vi "thrustAlloc.vi"(2 "tau":dbl[](array[numeric])) -> (5 "u_0":dbl, 6 "u_1":dbl, 7 "u_2":dbl)   [LabVIEW 2014]
uses:
  <vilib>/imath/engines/lvmath2/RunTimeEngine/Managers/WorkSpace/UID Generator.vi
  <vilib>/imath/engines/lvmath2/RunTimeEngine/ArithmeticOperatorToken/NIMS_ArithmeticOperator_multmx(M,CV).vi
  <instcachedir>/0/NIMS_ArithmeticOperator_multmx(M,CV)_787B4652E60B4C52835A7FB23671E425.lvgen/NIMS_ArithmeticOperator_multmx(M,CV)_787B4652E60B4C52835A7FB23671E425_000.vi
  <vilib>/imathl/engines/lvmath/Functions/Error Handling/Create Error.vi
  <vilib>/imath/engines/lvmath2/RunTimeEngine/IndexRead/NIMS M(S).vi
  <instcachedir>/0/NIMS M(S)_B826C018497E4940AE96BD27B540B6FB.lvgen/NIMS M(S)_B826C018497E4940AE96BD27B540B6FB_000.vi
  <vilib>/imath/engines/lvmath2/RunTimeEngine/BuiltInFunctions/diag/NIMS_diag.vi
  <instcachedir>/0/NIMS_diag_3C4F3DCE8A2D4541A558217542783B22.lvgen/NIMS_diag_3C4F3DCE8A2D4541A558217542783B22_003.vi
  <vilib>/imath/engines/lvmath2/RunTimeEngine/RunTimeType/NIMS_RunTimeType_From StrictType (excl LVString).vi
  <instcachedir>/0/NIMS_RunTimeType_From StrictType (excl LVString)_15A5391EEA9C4AACB9955AC755B83D29.lvgen/NIMS_RunTimeType_From StrictType (excl LVString)_15A5391EEA9C4AACB9955AC755B83D29_000.vi
  <vilib>/imath/engines/lvmath2/RunTimeEngine/LocalVariableDefStatement/MC_LocalVariableDefStatement_Display.vi
  <vilib>/imath/engines/lvmath2/RunTimeEngine/ArithmeticOperatorToken/NIMS_ArithmeticOperator_multmx.vi
  <instcachedir>/0/NIMS_ArithmeticOperator_multmx_CE3986B82B8C4E94A31593A7EF82383B.lvgen/NIMS_ArithmeticOperator_multmx_CE3986B82B8C4E94A31593A7EF82383B_004.vi
  <vilib>/imath/engines/lvmath2/RunTimeEngine/BuiltInFunctions/inv/NIMS_inv(GM).vi
  <instcachedir>/0/NIMS_inv(GM)_A6DF8FE880224208AACFE4CF9F659502.lvgen/NIMS_inv(GM)_A6DF8FE880224208AACFE4CF9F659502_000.vi
  <vilib>/imath/engines/lvmath2/RunTimeEngine/ErrorHandling/NIMS_Error From Error Code.vi
  <vilib>/imath/engines/lvmath2/RunTimeEngine/Managers/SymbolTable/Clear UID.vi
  <vilib>/imath/engines/lvmath2/RunTimeEngine/NodeEndStatement/NIMS_NodeEndStatement_Output.vi
  <instcachedir>/0/NIMS_NodeEndStatement_Output_53EC0D466D134D7ABD903AC30B43404B.lvgen/NIMS_NodeEndStatement_Output_53EC0D466D134D7ABD903AC30B43404B_002.vi
  <vilib>/imath/engines/lvmath2/RunTimeEngine/ErrorHandling/NIMS_Finalize Error.vi
  <vilib>/imath/engines/lvmath2/RunTimeEngine/ErrorHandling/NIMS_Create Error From Enums.vi
  <vilib>/imath/engines/lvmath2/RunTimeEngine/ArithmeticOperatorToken/NIMS_ArithmeticOperator_multmx-internal.vi
  <vilib>/imath/engines/lvmath2/RunTimeEngine/Managers/SymbolTable/NIMS_WorkSpace.lvlib
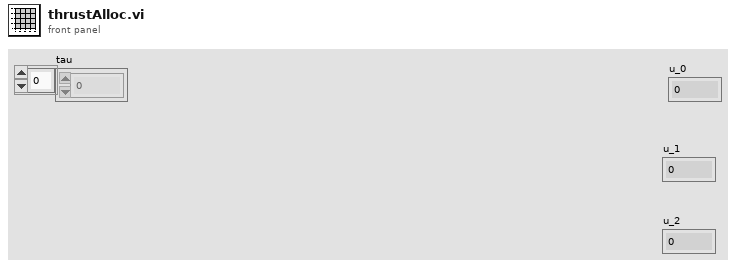
[diagram p1: front panel]
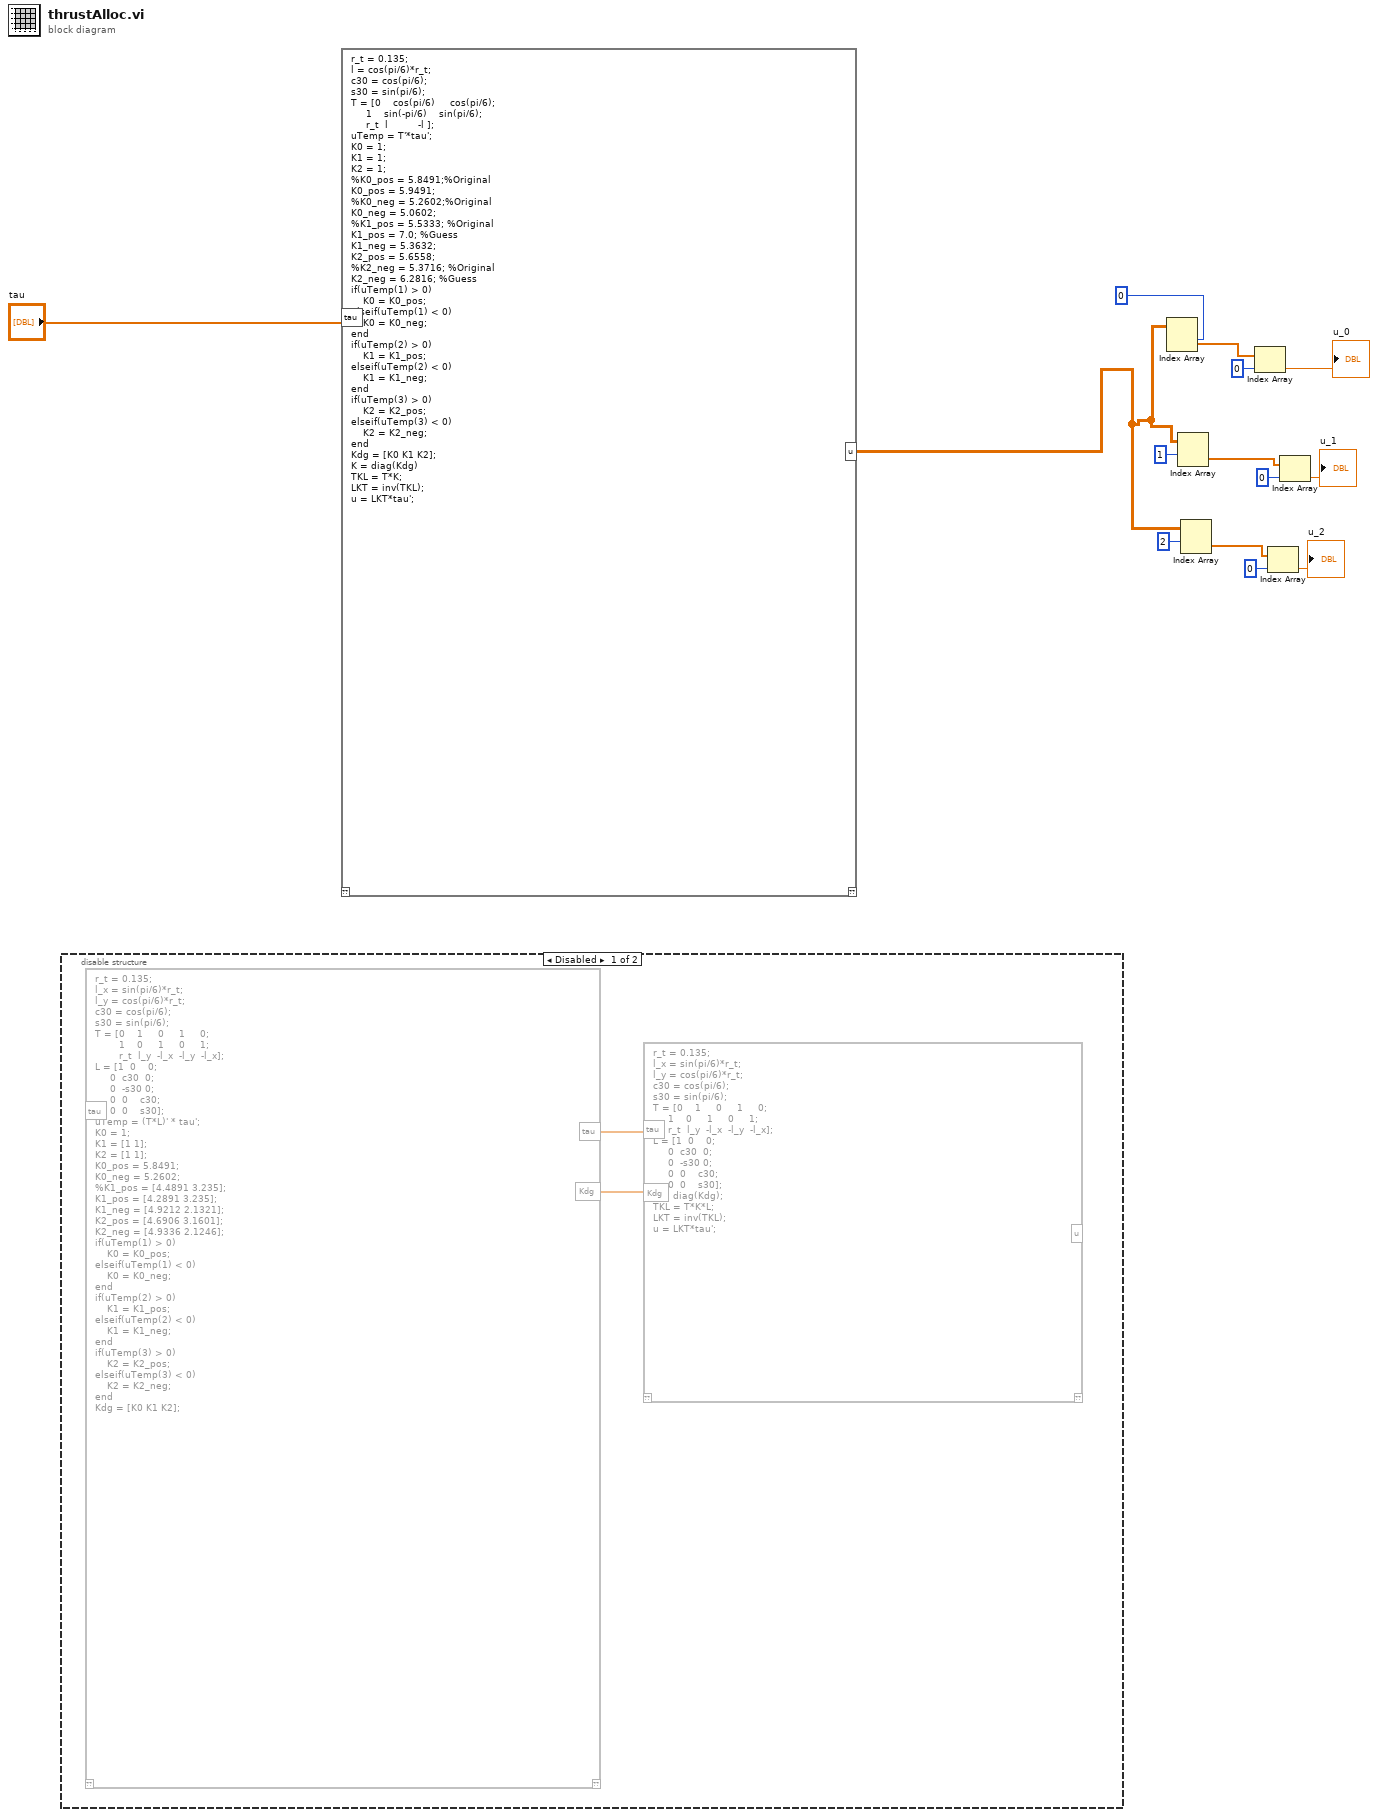
[diagram p0: block diagram]
diagram:
  n1 = disable-structure shown="Disabled" {
    frame Disabled {
      n2 = mathscript code="r_t = 0.135;\nl_x = sin(pi/6)*r_t;\nl_y = cos(pi/6)*r_t;\nc30 = cos(pi/6);\ns30 = sin(pi/6);\nT = [0    1     0     1     0;\n        1    0     1     0     1;\n        r_t  l_y  -l_x  -l_y  -l_x];\nL = [1  0    0;\n     0  c30  0;\n     0  -s30 0;\n     0  0    c30;\n     0  0    s30];\nuTemp = (T*L)' * tau';\nK0 = 1;\nK1 = [1 1];\nK2 = [1 1];\nK0_pos = 5.8491;\nK0_neg = 5.2602;\n%K1_pos = [4.4891 3.235];\nK1_pos = [4.2891 3.235];\nK1_neg = [4.9212 2.1321];\nK2_pos = [4.6906 3.1601];\nK2_neg = [4.9336 2.1246];\nif(uTemp(1) > 0)\n    K0 = K0_pos;\nelseif(uTemp(1) < 0)\n    K0 = K0_neg;\nend\nif(uTemp(2) > 0)\n    K1 = K1_pos;\nelseif(uTemp(2) < 0)\n    K1 = K1_neg;\nend\nif(uTemp(3) > 0)\n    K2 = K2_pos;\nelseif(uTemp(3) < 0)\n    K2 = K2_neg;\nend\nKdg = [K0 K1 K2];"() -> ("Kdg"=w16:dbl[], "tau"=w15:dbl[])  [unwired: 2 in, 1 out]
      n3 = mathscript code="r_t = 0.135;\nl_x = sin(pi/6)*r_t;\nl_y = cos(pi/6)*r_t;\nc30 = cos(pi/6);\ns30 = sin(pi/6);\nT = [0    1     0     1     0;\n     1    0     1     0     1;\n     r_t  l_y  -l_x  -l_y  -l_x];\nL = [1  0    0;\n     0  c30  0;\n     0  -s30 0;\n     0  0    c30;\n     0  0    s30];\nK = diag(Kdg);\nTKL = T*K*L;\nLKT = inv(TKL);\nu = LKT*tau';"("tau"=w15, "Kdg"=w16) -> ()  [unwired: 1 in, 2 out]
    }
    frame Enabled {
    }
  }
  n4 = mathscript code="r_t = 0.135;\nl = cos(pi/6)*r_t;\nc30 = cos(pi/6);\ns30 = sin(pi/6);\nT = [0    cos(pi/6)     cos(pi/6);\n     1    sin(-pi/6)    sin(pi/6);\n     r_t  l          -l ];\nuTemp = T'*tau'; \nK0 = 1;\nK1 = 1;\nK2 = 1;\n%K0_pos = 5.8491;%Original\nK0_pos = 5.9491;\n%K0_neg = 5.2602;%Original\nK0_neg = 5.0602;\n%K1_pos = 5.5333; %Original\nK1_pos = 7.0; %Guess\nK1_neg = 5.3632;\nK2_pos = 5.6558;\n%K2_neg = 5.3716; %Original\nK2_neg = 6.2816; %Guess\nif(uTemp(1) > 0)\n    K0 = K0_pos;\nelseif(uTemp(1) < 0)\n    K0 = K0_neg;\nend\nif(uTemp(2) > 0)\n    K1 = K1_pos;\nelseif(uTemp(2) < 0)\n    K1 = K1_neg;\nend\nif(uTemp(3) > 0)\n    K2 = K2_pos;\nelseif(uTemp(3) < 0)\n    K2 = K2_neg;\nend\nKdg = [K0 K1 K2];\nK = diag(Kdg)\nTKL = T*K;\nLKT = inv(TKL);\nu = LKT*tau';"("tau"="tau") -> ("u"=w1:dbl[][])  [unwired: 1 in, 1 out]
  n5 = Index Array(array=w1, index (row)=0) -> (element=w13:dbl[])  [unwired: 1 in]
  n6 = Index Array(array=w1, index (row)=1) -> (element=w9:dbl[])  [unwired: 1 in]
  n7 = Index Array(array=w1, index (row)=2) -> (element=w5:dbl[])  [unwired: 1 in]
  n8 = Index Array(array=w13, index=0) -> (element=→"u_0":dbl)
  n9 = Index Array(array=w5, index=0) -> (element=→"u_2":dbl)
  n10 = Index Array(array=w9, index=0) -> (element=→"u_1":dbl)
